vi "Configure923xAcquisition.vi"(8 "error in (no error)":errorcluster) -> (0 "error out":errorcluster, 2 "register data sets":T1[](array[typedef]), 3 "923x Acquisition Config":T4={"Acq"=FALSE, "NumberOfModules"=0, "Dynamic FPGA VI Ref"=refnum, "KeyphasorX3"=[], "FixedSizeX32"={"EnabledChannels"=[], "Sensitivity"=[], "InputConfig"=[]}, "SamplingInfo"={"Number of Channels"=4, "Sampling Rate"=4.0, "Channels"=[], "Units"=[], "Offsets"=[]}, "Normal Mode Sample Rate"=0.0, "BlockSize (sec)"=0.0, "Samples To Read (per chan)"=0, "RunningAcquisitionLength"=0.0, "Settling Time"=0.0, "Fpga Tach Buffer Size (samples)"=0, "Waveform Groups"=[], "Acquisition Block Number"=0, "Device Name"="", "ValidConfig"=FALSE, "Last Dynamic Module"="", "HighPassFilterState"=[], "Low Frequency Cutoff"=[], "BurstMode"={"Acquisition Time"=0.0, "Sample Rate"=0.0, "Collection Reason"=""}} {"HighPassFilterState"."Filter State" format="%.2f"; "HighPassFilterState"."IIR Filter Cluster"."Forward Coefficients" format="%.2f"; "HighPassFilterState"."IIR Filter Cluster"."Reverse Coefficients" format="%.2f"; "FixedSizeX32"."InputConfig" items=["AC Coupled", "DC Coupled", "IEPE AC Coupled"]}, 5 "valid":bool)   [LabVIEW 2017, in "CmsAcquisition.lvlib"]
uses:
  <vilib>/addons/InsightCM/Devices/Shared/Cms/CmsAcquisition/CmsAcquisition.lvlib
  <vilib>/addons/InsightCM/Devices/Shared/Cms/CmsAcquisition/controls/Configuration.ctl
  <vilib>/addons/InsightCM/Devices/Shared/Cms/CmsAcquisition/controls/TachometerConfig.ctl
  <vilib>/addons/InsightCM/Devices/Shared/Cms/CmsAcquisition/controls/FixedSizeArrays.ctl
  <vilib>/LabVIEW Targets/FPGA/cRIO/shared/nicrio_ModuleControls/nicrio_cRIO-9232_ConfigModeRing.ctl
  <vilib>/addons/InsightCM/Devices/Shared/Cms/cRIOWfmAcq/subVIs/RIO Wfm Cust Ctrls/rwfm_SamplingInfo.ctl
  <vilib>/addons/InsightCM/Devices/Shared/Cms/CmsAcquisition/controls/Group.ctl
  <vilib>/addons/InsightCM/Devices/Shared/Cms/CmsAcquisition/controls/Channel.ctl
  <vilib>/addons/InsightCM/Utilities/Analysis/Vibration/controls/HighPassFilterState.ctl
  <vilib>/addons/InsightCM/Devices/Shared/Cms/CmsAcquisition/controls/BurstMode.ctl
  <vilib>/addons/InsightCM/Devices/Shared/Common/DataEventCreator/controls/RegisterDataSets.ctl
  <vilib>/addons/InsightCM/Devices/Shared/Cms/CmsDataEventCreator/controls/DataSetRegistry.ctl
  <vilib>/addons/InsightCM/Devices/Shared/Common/DataEvent/controls/DataSetType.ctl
  <vilib>/addons/InsightCM/Utilities/GlobalConfiguration/GlobalConfiguration.lvlib
  <vilib>/addons/InsightCM/Devices/Shared/Cms/cRIOWfmAcq/cRIOWfmLib.lvlib
  <vilib>/addons/InsightCM/Devices/Shared/Common/DataEvent/DataEvent.lvlib
  <vilib>/addons/InsightCM/Devices/Shared/Cms/CmsDataEventCreator/CmsDataEventCreator.lvlib
  <vilib>/addons/InsightCM/Devices/Shared/Common/DataEventCreator/DataEventCreator.lvlib
  <vilib>/addons/InsightCM/Utilities/Analysis/Vibration/VibrationAnalysisFunctions.lvlib
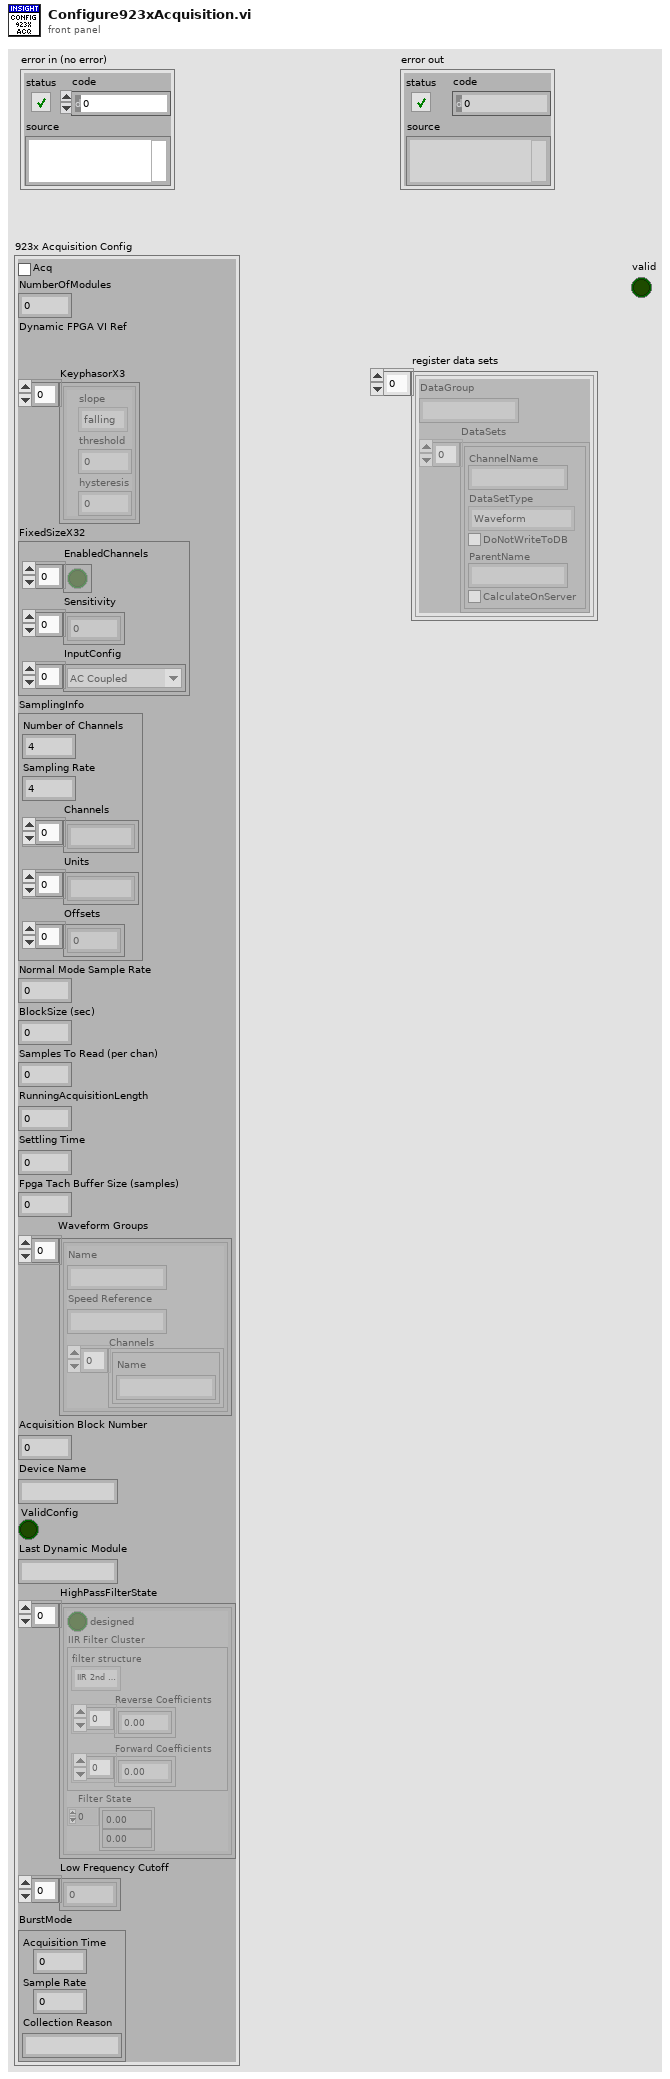
[diagram p1: front panel]
types:
  T1 = typedef "DataEventCreator.lvlib/RegisterDataSets.ctl" = cluster{"DataGroup":string, "DataSets":T2[]}
  T2 = typedef "CmsDataEventCreator.lvlib/DataSetRegistry.ctl" = cluster{"ChannelName":string, "DataSetType":T3, "DoNotWriteToDB":bool, "ParentName":string, "CalculateOnServer":bool}
  T3 = typedef "DataEvent.lvlib/DataSetType.ctl" = enum16{"Waveform", "SpeedProfile", "ThermalImage", "EmsaSweep"}
  T4 = typedef "CmsAcquisition.lvlib/Configuration.ctl" = cluster{"Acq":bool, "NumberOfModules":i16, "Dynamic FPGA VI Ref":refnum<k20>, "KeyphasorX3":T5[], "FixedSizeX32":T6, "SamplingInfo":T8, "Normal Mode Sample Rate":dbl, "BlockSize (sec)":dbl, "Samples To Read (per chan)":i32, "RunningAcquisitionLength":dbl, "Settling Time":dbl, "Fpga Tach Buffer Size (samples)":i32, "Waveform Groups":T9[], "Acquisition Block Number":i32, "Device Name":string, "ValidConfig":bool, "Last Dynamic Module":string, "HighPassFilterState":T11[], "Low Frequency Cutoff":dbl[], "BurstMode":T12}
  T5 = typedef "CmsAcquisition.lvlib/TachometerConfig.ctl" = cluster{"slope":enum16{"falling", "rising"}, "threshold":dbl, "hysteresis":dbl}
  T6 = typedef "CmsAcquisition.lvlib/FixedSizeArrays.ctl" = cluster{"EnabledChannels":bool[], "Sensitivity":dbl[], "InputConfig":T7[]}
  T7 = typedef "nicrio_cRIO-9232_ConfigModeRing.ctl" = u8
  T8 = typedef "cRIOWfmLib.lvlib/rwfm_SamplingInfo.ctl" = cluster{"Number of Channels":i32, "Sampling Rate":dbl, "Channels":string[], "Units":string[], "Offsets":sgl[]}
  T9 = typedef "CmsAcquisition.lvlib/Group.ctl" = cluster{"Name":string, "Speed Reference":string, "Channels":T10[]}
  T10 = typedef "CmsAcquisition.lvlib/Channel.ctl" = cluster{"Name":string}
  T11 = typedef "VibrationAnalysisFunctions.lvlib/HighPassFilterState.ctl" = cluster{"designed":bool, "IIR Filter Cluster":cluster{"filter structure":enum32{"IIR 2nd Order", "IIR 4th Order"}, "Reverse Coefficients":dbl[], "Forward Coefficients":dbl[]}, "Filter State":dbl[]}
  T12 = typedef "CmsAcquisition.lvlib/BurstMode.ctl" = cluster{"Acquisition Time":dbl, "Sample Rate":dbl, "Collection Reason":string}
  T13 = typedef "R2_Device.ctl" = cluster{"Id":string, "Name":string, "DeviceType":string, "HardwareName":string, "IpAddress":string, "HardwareInfo":T14[], "ApplicationType":string, "ApplicationVersion":string, "EquipmentIds":string[], "ConfigurationVersion":string, "State":T15, "Properties":T14[], "DataGroups":T16[], "BurstModeTrigger":T20}
  T14 = typedef "KeyValuePair.ctl" = cluster{"Key":string, "Value":string}
  T15 = typedef "DeviceState.ctl" = cluster{"Disabled":bool}
  T16 = typedef "R2_DataGroup.ctl" = cluster{"Name":string, "OperatingStates":T17[], "Properties":T14[], "EquipmentIds":string[], "AssetNodeId":string}
  T17 = typedef "OperatingState.ctl" = cluster{"Name":string, "Properties":T14[], "Triggers":T18[]}
  T18 = typedef "Trigger.ctl" = cluster{"Type":string, "Expression":string, "Conditions":T19[]}
  T19 = typedef "Condition.ctl" = cluster{"Source":string, "Type":string, "Operator":string, "CompareTo":string, "DwellSeconds":dbl}
  T20 = typedef "BurstModeTrigger.ctl" = cluster{"Trigger":T18, "SampleRate":string, "AcquisitionLength":string}
  T21 = typedef "R2_Channel.ctl" = cluster{"Id":string, "DeviceId":string, "Name":string, "ChannelType":string, "HardwareKey":string, "HardwareChannel":string, "DataGroup":string, "Keywords":string[], "EquipmentIds":string[], "Properties":T14[], "Metrics":T22[], "AssetNodeId":string, "MeasType":string, "AssetName":string}
  T22 = typedef "Metric.ctl" = cluster{"Id":string, "Name":string, "Unit":string, "Properties":T14[], "MetricDefinitionInstanceId":string}
  T23 = typedef "SectionKeyValues.ctl" = cluster{"Section":string, "KeyValues":T14[]}
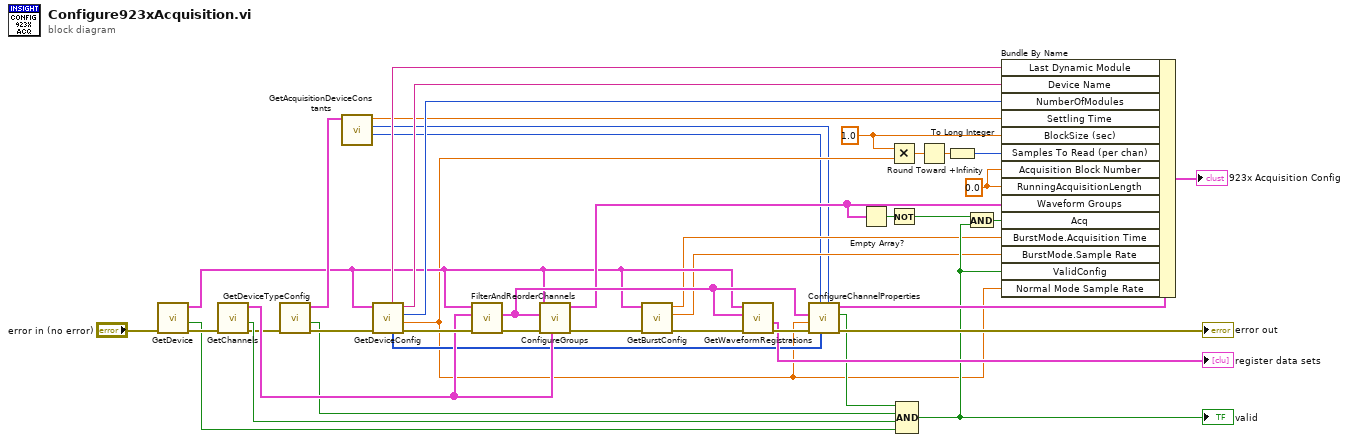
[diagram p0: block diagram]
diagram:
  w15 = 0.0 ("RunningAcquisitionLength")
  w37 = 1.0 ("Block Size (sec)")
  n1 = call <vilib>:"GetDevice.vi"("error in (no error)"="error in (no error)") -> ("error out"=w40:errorcluster, "found"=w26:bool, "device configuration"=w9:T13)  [unwired: 8 in]
  n2 = call <vilib>:"GetChannels.vi"("error in (no error)"=w40) -> ("error out"=w18:errorcluster, "found"=w25:bool, "channels"=w27:T21[])  [unwired: 8 in]
  n3 = call <vilib>:"GetDeviceTypeConfig.vi"("error in (no error)"=w18) -> ("error out"=w24:errorcluster, "found"=w22:bool, "key values"=w23:T23[])  [unwired: 8 in]
  n4 = call <vilib>:"GetAcquisitionDeviceConstants.vi"("key values"=w23) -> ("fpga tach buffer minimum"=w1:i32, "fpga tach buffer multiplier"=w2:i32, "settling time (seconds)"=w4:dbl)  [unwired: 8 in]
  n5 = call <vilib>:"GetDeviceConfig.vi"("error in (no error)"=w24, "Device"=w9) -> ("error out"=w33:errorcluster, "Sample Rate"=w3:dbl, "Number of Dynamic Modules"=w35:i32, "Name"=w29:string, "Channels per Dynamic Module"=w20:i32[], "Last Dynamic Module"=w19:string)  [unwired: 4 in]
  n6 = call <vilib>:"FilterAndReorderChannels.vi"("error in (no error)"=w33, "channels"=w27, "device"=w9) -> ("error out"=w31:errorcluster, "acquisition channels (in acquisition order)"=w28:T21[])  [unwired: 7 in]
  n7 = call <vilib>:"ConfigureGroups.vi"("all channels"=w27, "error in (no error)"=w31, "acquisition channels (in acquisition order)"=w28, "device"=w9) -> ("error out"=w8:errorcluster, "groups"=w14:T9[])  [unwired: 6 in]
  n8 = call <vilib>:"GetBurstConfig.vi"("error in (no error)"=w8, "device configuration"=w9) -> ("error out"=w7:errorcluster, "burst sample rate"=w5:dbl, "burst acq length"=w6:dbl)  [unwired: 7 in]
  n9 = call <vilib>:"GetWaveformRegistrations.vi"("error in (no error)"=w7, "acquisition channels (in acquisition order)"=w28, "device"=w9) -> ("error out"=w30:errorcluster, "register data sets"=→"register data sets":T1[])  [unwired: 7 in]
  n10 = call <vilib>:"ConfigureChannelProperties.vi"("fpga tach buffer multiplier"=w2, "Channels per Dynamic Module"=w20, "fpga tach buffer minimum"=w1, "error in (no error)"=w30, "Sampling Rate"=w3, "Filtered Channels (in acquisition order)"=w28) -> ("error out"=→"error out":errorcluster, "valid"=w16:bool, "acq config"=w17:T4)  [unwired: 3 in]
  n11 = Empty Array?(array=w14) -> (empty?=w13:bool)
  n12 = Multiply(x=w37, y=w3) -> (x*y=w39:dbl)
  n13 = Not(x=w13) -> (.not. x?=w12:bool)
  n14 = Compound Arithmetic op=AND(w16, w22, w25, w26) -> (w10:bool)
  "valid" <- w10
  n15 = Round Toward +Infinity(x=w39) -> (ceil(x): smallest int >= x=w38:dbl)
  n16 = To Long Integer(number=w38) -> (32bit integer=w36:i32)
  n17 = And(x=w12, y=w10) -> (x .and. y?=w11:bool)
  n18 = Bundle By Name(cluster=w17, "Last Dynamic Module"=w19, "Device Name"=w29, "NumberOfModules"=w35, "Settling Time"=w4, "BlockSize (sec)"=w37, "Samples To Read (per chan)"=w36, "Acquisition Block Number"=w15, "RunningAcquisitionLength"=w15, "Waveform Groups"=w14, "Acq"=w11, "BurstMode.Acquisition Time"=w6, "BurstMode.Sample Rate"=w5, "ValidConfig"=w10, "Normal Mode Sample Rate"=w3) -> (→"923x Acquisition Config":T4)
